vi "test.vi"() -> ()   [LabVIEW 2011]
panel:
  in  "Choose Address":refnum<visa-resource-name>="ASRL1::INSTR"
  in  "Command":string
  out "Response":string
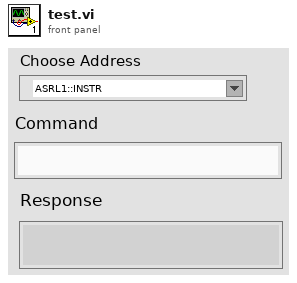
[diagram p1: front panel]
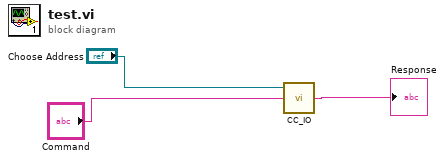
[diagram p0: block diagram]
diagram:
  n1 = call "CC_IO.vi"("Output Command"="Command", "VISA In"="Choose Address") -> ("Input String"=→"Response":string)  [unwired: 1 in, 2 out]
